vi "Send move to stages.vi"(8 "error in (no error)":errorcluster, 11 "ImageStack in":refnum<class "ImageStack.lvclass">) -> (0 "error out":errorcluster, 3 "ImageStack out":refnum<class "ImageStack.lvclass">)   [LabVIEW 2012, in "ImageStack.lvclass"]
uses:
  ImageStack.lvclass
  <vilib>/Distrio/Murmex/GenericMessage/GenericMessage.lvclass
  ImageStack.lvclass/ImageStack.ctl
  <vilib>/Distrio/Murmex/Message/Message.lvclass
  <vilib>/Distrio/Murmex/Murmex/Murmex.lvclass
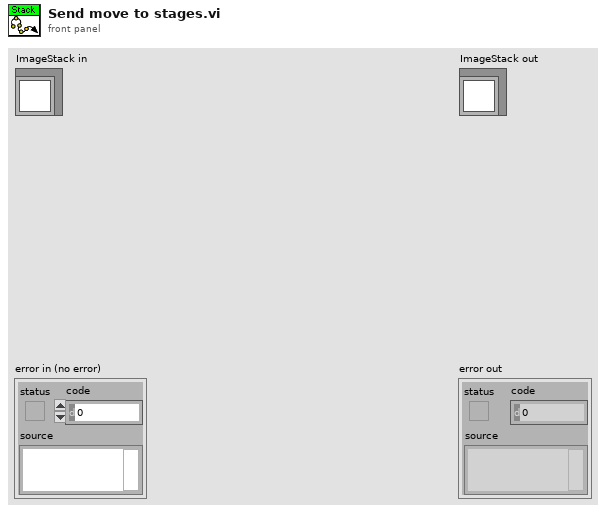
[diagram p1: front panel]
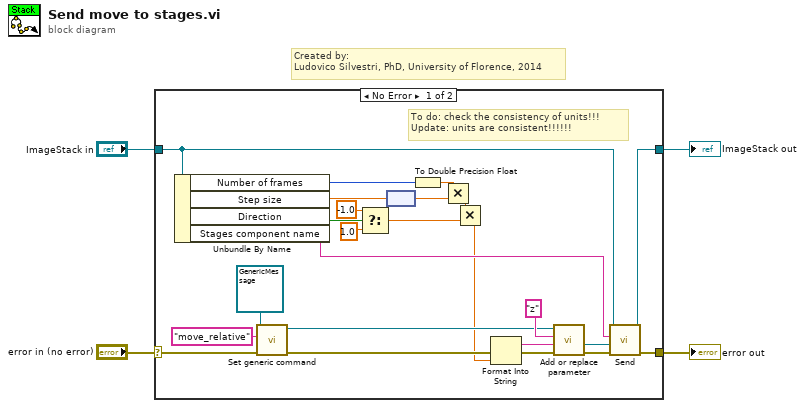
[diagram p0: block diagram]
diagram:
  # "Created by:\nLudovico Silvestri, PhD, University of Florence, 2014"
  n1 = case shown="No Error" "error in (no error)" {
    selector: "error in (no error)" -> [w26 w30]
    tunnel: [w16 w30] -> w3
    tunnel: [w14 w29] -> w1
    tunnel: "ImageStack in" -> [w15 w29]
    frame No Error {
      # "To do: check the consistency of units!!!\nUpdate: units are consistent!!!!!!"
      n2 = Unbundle By Name(w15) -> ("Number of frames"=w24:u16, "Step size"=w25:dbl[unit], "Direction"=w11:bool, "Stages component name"=w12:string)
      n3 = call <vilib>:"Set generic command.vi"("error in (no error)"=w26, "generic command"="move_relative" ("command string"), "GenericMessage in"=refnum<class "GenericMessage.lvclass"> refnum ("Murmex.lvlib:GenericMessage")) -> ("error out"=w22:errorcluster, "GenericMessage out"=w18:refnum<class "GenericMessage.lvclass">)  [unwired: 7 in]
      n4 = Select(t=-1.0 ("y"), s=w11, f=1.0 ("y")) -> (s? t:f=w8:dbl)
      n5 = node(w25) -> (w5:dbl)
      n6 = To Double Precision Float(number=w24) -> (double precision float=w23:dbl)
      n7 = Multiply(x=w23, y=w5) -> (x*y=w7:dbl)
      n8 = Multiply(x=w7, y=w8) -> (x*y=w6:dbl)
      n9 = Format Into String(error in=w22, w6) -> (resulting string=w20:string, error out=w21:errorcluster)  [unwired: 2 in]
      n10 = call <vilib>:"Add or replace parameter.vi"("error in (no error)"=w21, "value"=w20, "name"="z", "Message in"=w18) -> ("error out"=w17:errorcluster, "Message out"=w13:refnum<class "GenericMessage.lvclass">)  [unwired: 6 in]
      n11 = call <vilib>:"Send.vi"("error in (no error)"=w17, "Message"=w13, "recipient"=w12, "Murmex in"=w15) -> ("error out"=w16:errorcluster, "Murmex out"=w14:refnum<class "ImageStack.lvclass">)  [unwired: 6 in]
    }
    frame Error {
    }
  }
  "error out" <- w3
  "ImageStack out" <- w1
